vi "Instrument.LogPGSQL.vi"(6 "Deprecated":bool, 8 "error in (no error)":errorcluster, 9 "Data":variant=variant(bool FALSE), 10 "Paths":string, 11 "Instrument":refnum<class "Instrument.lvclass">) -> (0 "error out":errorcluster, 3 "Instrument out":refnum<class "Instrument.lvclass">)   [LabVIEW 2019, in "Instrument.lvlib" / "Instrument.lvclass"]
doc: "Deprecated in favor of Instrument.logToDatabase.vi"
uses:
  Instrument.lvclass
panel:
  # "For instructions on how to use the JKI State Machine Objects, examples and video tutorials, visit:\nhttp://jki.net/state-machine-objects/\n\nJKI State Machine Objects™\nhttp://jki.net/state-machine-objects/\nCopyright (C) 2005-2015, JKI <info@jki.net>\nALL RIGHTS RESERVED"
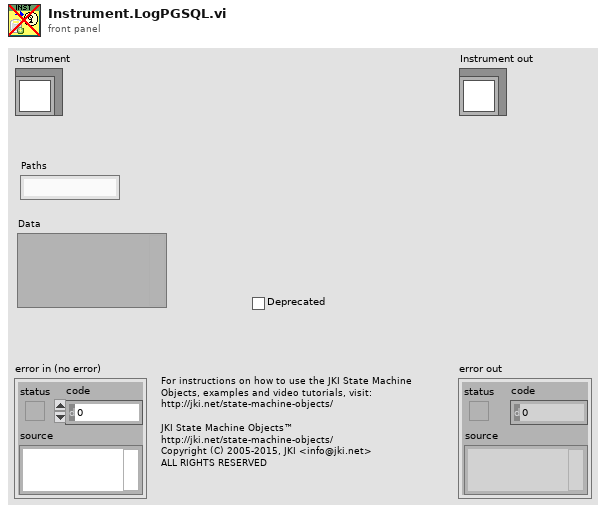
[diagram p1: front panel]
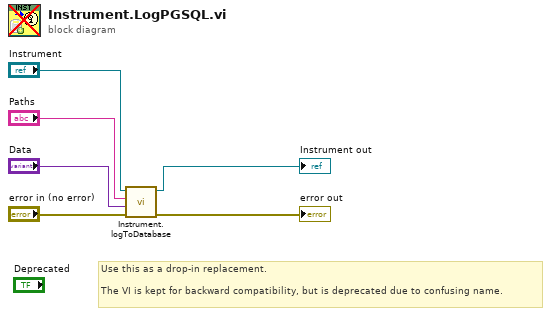
[diagram p0: block diagram]
diagram:
  # "Use this as a drop-in replacement.\n\nThe VI is kept for backward compatibility, but is deprecated due to confusing name."
  n1 = call "Instrument.logToDatabase.vi"("error in (no error)"="error in (no error)", "Data"="Data", "Paths"="Paths", "Instrument"="Instrument") -> ("error out"=→"error out":errorcluster, "Instrument out"=→"Instrument out":refnum<class "Instrument.lvclass">)  [unwired: 6 in]
